vi "PH_SHS_Analysis_Calibrator.get Text for Save Result Dialog.vi"(0 "i ref in":refnum<vi>, 5 "error in (no error)":errorcluster) -> (14 "i ref out":refnum<vi>, 17 "User Dialog":string, 19 "error out":errorcluster)   [LabVIEW 2014, in "PH_SHS_Analysis_Calibrator.lvlib"]
doc: "Thi VI checks whether all data are taken with sucess to set the User Dialog."
uses:
  PH_SHS_Analysis_Calibrator.lvlib
  PH_Basics/PH_Img_BaseClass/PH_Img_BaseClass.lvlib
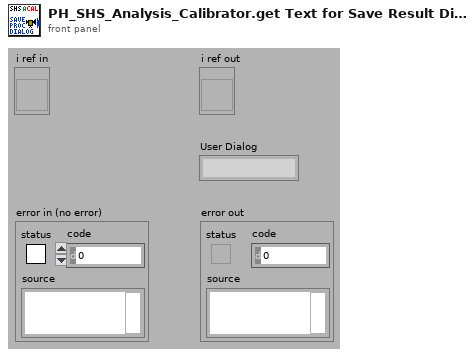
[diagram p1: front panel]
types:
  T1 = typedef "PH_SHS_Analysis_Calibrator.lvlib/PH_SHS_Analysis_Calibrator.i attribute.ctl" = cluster{"GUI Refs":cluster{"Available Cams":refnum<vi>, "OK":refnum<vi>, "Skip":refnum<vi>, "Repeat":refnum<vi>, "Cancel":refnum<vi>, "Dialog":refnum<vi>, "Enough Images?":refnum<vi>}, "Cam instances":string[], "Status":cluster{"#":i32, "Data calculated":bool, "Wanted #":i32}, "IMAQ Image Array":T2[], "Pixel Size [µm]":dbl, "MLA Pitch [µm]":dbl, "Method":enum16{"automatic", "manual"}, "Enough Images?":bool, "SHS Reference Result":T3, "Calculation Error":errorcluster}
  T2 = typedef "IMAQ Image.ctl" = refnum<image>
  T3 = typedef "SHS_Common.lvlib/SHSReference.ctl" = cluster{"Reference":T4[][], "Lens Array Pitch [px]":dbl}
  T4 = typedef "SHS_Common.lvlib/ReferencePoint.ctl" = cluster{"Rect":T5, "Point":T6}
  T5 = typedef "SHS_Common.lvlib/Rectangle.ctl" = cluster{"Left":i32, "Top":i32, "Right":i32, "Bottom":i32}
  T6 = typedef "SHS_Common.lvlib/Point.ctl" = cluster{"x":dbl, "y":dbl, "valid?":bool, "weight":dbl}
  T7 = typedef "PH_Img_BaseClass.lvlib/PH_Img_BaseClass.i attribute.ctl" = cluster{"GUI Refs":T8, "Timeout Image [ms]":i32, "Default Periodic Period [ms]":i32, "Camera":cluster{"Instancename":string, "Notifier":refnum<notifier>}, "Palette":T9, "Cam Settings":cluster{"Cam ID":string, "Gain":dbl, "Brightness":dbl, "Shutter":dbl, "Cam Info Failure":bool, "Mode":i32}}
  T8 = typedef "PH_Img_BaseClass.lvlib/PH_Img_BaseClass.GUI Refs.ctl" = cluster{"Timeout":refnum<vi>, "Image":refnum<vi>, "Palette":refnum<vi>, "Timeout Set":refnum<vi>}
  T9 = typedef "PH_Img_BaseClass.lvlib/PH_Img_BaseClass.Palette.ctl" = i32
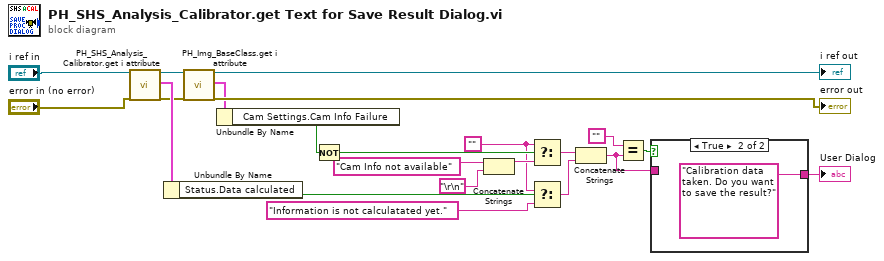
[diagram p0: block diagram]
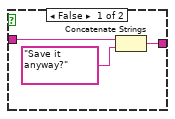
[diagram p2: hidden frame]
diagram:
  w15 = ""
  n1 = call "PH_SHS_Analysis_Calibrator.get i attribute.vi"("i ref in"="i ref in", "error in (no error)"="error in (no error)") -> ("i ref out"=w21:refnum<vi>, "i attribute"=w19:T1, "error out"=w4:errorcluster)  [unwired: 15 in]
  n2 = Unbundle By Name(w19) -> ("Status.Data calculated"=w7:bool)
  n3 = call "PH_Img_BaseClass.get i attribute.vi"("i ref in"=w21, "error in (no error)"=w4) -> ("i ref out"=→"i ref out":refnum<vi>, "i attribute"=w2:T7, "error out"=→"error out":errorcluster)  [unwired: 15 in]
  n4 = Unbundle By Name(w2) -> ("Cam Settings.Cam Info Failure"=w1:bool)
  n5 = Not(x=w1) -> (.not. x?=w18:bool)
  n6 = Concatenate Strings("Cam Info not available", "\r\n") -> (w16:string)
  n7 = Select(t=w15, s=w18, f=w16) -> (s? t:f=w13:string)
  n8 = Select(t=w15, s=w7, f="Information is not calculatated yet.") -> (s? t:f=w12:string)
  n9 = Concatenate Strings(w13, w12) -> (w8:string)
  n10 = Equal?(x="" ("y"), y=w8) -> (x = y?=w11:bool)
  n11 = case shown="True" w11 {
    tunnel: [w25 "Calibration data taken. Do you want to save the result?"] -> w9
    tunnel: w8 -> [w23 _]
    frame False {
      n12 = Concatenate Strings(w23, "Save it anyway?") -> (w25:string)
    }
    frame True {
    }
  }
  "User Dialog" <- w9
